vi "DFD FXP LabVIEW Code Generator_OBS_v75.vi"(7 "open FP? (F)":bool, 8 "error in (no error)":errorcluster, 9 "VI path":path, 10 "code type":T1(ring), 11 "filter in":T2={"mSRate_Fs"=1.0, "mSRate_Version"="1.0", "mSRate_Comments"="", "mSRate_OrgCoef"={"type"=enum."Undefined", "gain"=1.0, "coef a (k)"=[], "coef b (v)"=[]}, "mSRate_CurCoef"={"type"=enum."Undefined", "gain"=1.0, "coef a (k)"=[], "coef b (v)"=[]}, "mSRate_Quantized?"=FALSE, "mSRate_QCoef"={"type"=enum."Undefined", "gain"=1.0, "coef a (k)"=[], "coef b (v)"=[]}, "mSRate_QSettings"=[], "mSRate_Order"=0, "mSRate_Scaling"={"mSRate_ScaleByPowerOf2?"=FALSE, "mSRate_ScaleType"=enum."No Norm"}} {"mSRate_QSettings"."source" items=["Coef a/k"=0, "Coef b/v"=7, "Input"=1, "Output"=2, "Multiplicand"=3, "Product"=4, "Sum"=5, "Delay"=6, "Gain"=8]}) -> (0 "error out":errorcluster, 1 "dup VI path":path)   [LabVIEW 2017, in "NI_DigFilterLicensed.lvlib"]
doc: "Generates only fixed-point integer code for a fixed-point filter, without generating floating-point code. You can use this polymorphic VI to generate LabVIEW code or C code. You can select the polymorphic instance manually."
uses:
  <vilib>/addons/Digital Filter Design/NI_DigFilterLicensed.lvlib
  <vilib>/addons/Digital Filter Design/_Objects.llb/DFD Filter Obj.ctl
  <vilib>/addons/Digital Filter Design/_Objects.llb/DFD Filter Coef.ctl
  <vilib>/addons/Digital Filter Design/_Objects.llb/DFD Filter Structure Type Selector.ctl
  <vilib>/addons/Digital Filter Design/_Objects.llb/dfd_Internal Quantization Settings.ctl
  <vilib>/addons/Digital Filter Design/_Objects.llb/dfd_Internal Quantization Srcs.ctl
  <vilib>/addons/Digital Filter Design/_Objects.llb/DFD Coef Norm Type.ctl
  <vilib>/addons/Digital Filter Design/CodeGen.llb/DFD FXP Integer LabVIEW Code Generator.vi
  <vilib>/addons/Digital Filter Design/CodeGen.llb/DFD FXP LabVIEW FPGA Code Generator.vi
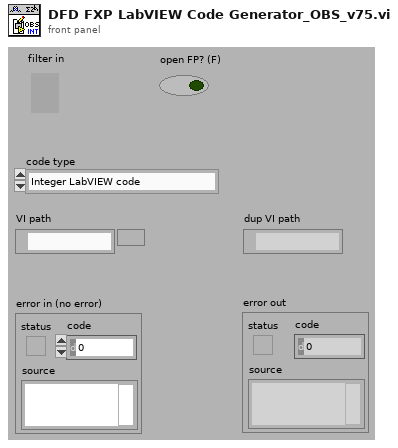
[diagram p1: front panel]
types:
  T1 = enum16{"Integer LabVIEW code", "SCTL-Optimized LabVIEW FPGA code"}
  T2 = typedef "NI_DigFilterLicensed.lvlib/DFD Filter Obj.ctl" = cluster{"mSRate_Fs":dbl, "mSRate_Version":string, "mSRate_Comments":string, "mSRate_OrgCoef":T3, "mSRate_CurCoef":T3, "mSRate_Quantized?":bool, "mSRate_QCoef":T3, "mSRate_QSettings":T5[], "mSRate_Order":i32, "mSRate_Scaling":cluster{"mSRate_ScaleByPowerOf2?":bool, "mSRate_ScaleType":T7}}
  T3 = typedef "NI_DigFilterLicensed.lvlib/DFD Filter Coef.ctl" = cluster{"type":T4, "gain":dbl, "coef a (k)":dbl[], "coef b (v)":dbl[]}
  T4 = typedef "NI_DigFilterLicensed.lvlib/DFD Filter Structure Type Selector.ctl" = enum16{"Undefined", "FIR Direct Form", "FIR Direct Form Transposed", "FIR Symmetric", "FIR Antisymmetric", "IIR Direct Form I", "IIR Direct Form I Transposed", "IIR Direct Form II", "IIR Direct Form II Transposed", "IIR Cascaded Second Order Sections Form I", "IIR Cascaded Second Order Sections Form I Transposed", "IIR Cascaded Second Order Sections Form II", "IIR Cascaded Second Order Sections Form II Transposed", "Lattice Allpass (basic sections)", "Lattice Allpass (one multiplier sections)", "Lattice Allpass (normalized sections)", "Lattice AR (basic sections)", "Lattice AR (one multiplier sections)", "Lattice AR (normalized sections)", "Lattice MA (minimum phase)", "Lattice MA (maximum phase)", "Lattice ARMA (basic sections)", "Lattice ARMA (one multiplier sections)", "Lattice ARMA (normalized sections)"}
  T5 = typedef "NI_DigFilterLicensed.lvlib/dfd_Internal Quantization Settings.ctl" = cluster{"source":T6, "wl":i16, "iwl":i16, "overflow mode":enum16{"Saturation", "Wrap"}, "rounding mode":enum16{"Nearest", "Truncation"}, "signed?":bool}
  T6 = typedef "NI_DigFilterLicensed.lvlib/dfd_Internal Quantization Srcs.ctl" = u16
  T7 = typedef "NI_DigFilterLicensed.lvlib/DFD Coef Norm Type.ctl" = enum16{"No Norm", "Time Domain 1-Norm", "Time Domain 2-Norm", "Time Domain Inf-Norm"}
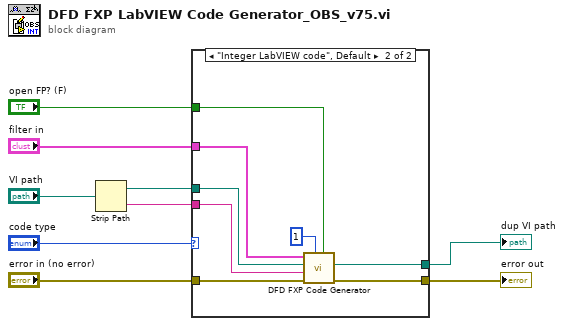
[diagram p0: block diagram]
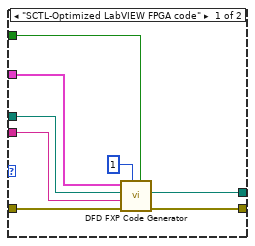
[diagram p2: hidden frame]
diagram:
  n1 = Strip Path(path="VI path") -> (stripped path=w7:path, name=w6:string)
  n2 = case shown="\"Integer LabVIEW code\", Default" "code type" {
    tunnel: w7 -> [w15 w23]
    tunnel: w6 -> [w16 w24]
    tunnel: "error in (no error)" -> [w17 w25]
    tunnel: "filter in" -> [w14 w22]
    tunnel: "open FP? (F)" -> [w13 w21]
    tunnel: [w11 w19] -> w2
    tunnel: [w10 w18] -> w1
    frame "SCTL-Optimized LabVIEW FPGA code" {
      n3 = call-poly <vilib>:"DFD FXP Code Generator.vi"("open project? (F)"=w13, "# channels"=1, "error in (no error)"=w17, "filter name"=w16, "destination folder"=w15, "filter in"=w14) -> ("error out"=w11:errorcluster, "lvproj path"=w10:path)  [unwired: 1 in, 3 out]
    }
    frame "Integer LabVIEW code", Default {
      n4 = call-poly <vilib>:"DFD FXP Code Generator.vi"("open project? (F)"=w21, "# channels"=1, "error in (no error)"=w25, "filter name"=w24, "destination folder"=w23, "filter in"=w22) -> ("error out"=w19:errorcluster, "lvproj path"=w18:path)  [unwired: 1 in, 3 out]
    }
  }
  "error out" <- w2
  "dup VI path" <- w1
